vi "Write SV.vi"(8 "error in (no error)":errorcluster, 10 "Data":dbl[](array[numeric]), 11 "Write Refs by Type":T1) -> (0 "error out":errorcluster)   [LabVIEW 2016, in "Shared Variable Interface.lvlib"]
uses:
  Shared Variable Interface.lvlib
  DataTypes/DBL.lvlib
  DataTypes/Bool.lvlib
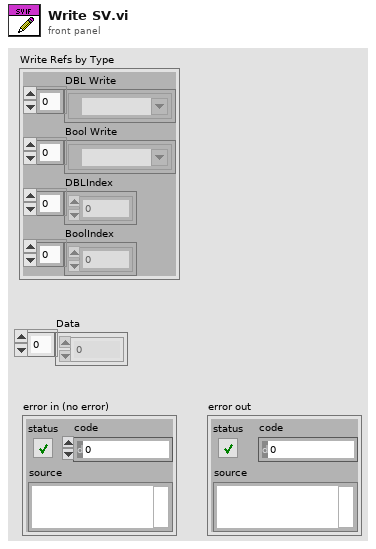
[diagram p1: front panel]
types:
  T1 = cluster{"DBL Write":refnum<k21>[], "Bool Write":refnum<k21>[], "DBLIndex":i32[], "BoolIndex":i32[]}
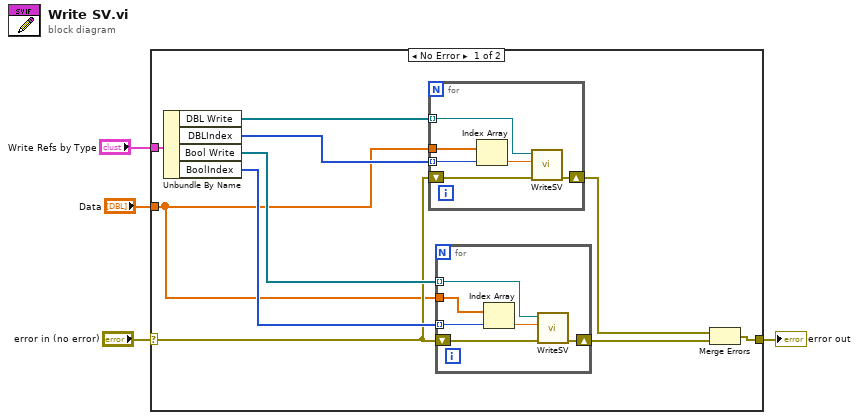
[diagram p0: block diagram]
diagram:
  n1 = case shown="No Error" "error in (no error)" {
    selector: "error in (no error)" -> [w7 w27]
    tunnel: [w14 w27] -> w4
    tunnel: "Data" -> [w6 _]
    tunnel: "Write Refs by Type" -> [w5 _]
    frame No Error {
      n2 = Unbundle By Name(w5) -> ("DBL Write"=w13:refnum<k21>[], "DBLIndex"=w12:i32[], "Bool Write"=w11:refnum<k21>[], "BoolIndex"=w10:i32[])
      n3 = for {
        tunnel: w13 -> [w21] mode=indexing
        tunnel: w12 -> [w26] mode=indexing
        shift-right: [w24] -> w8
        shift-left: w7 -> [w25]
        tunnel: w6 -> [w23]
        n4 = Index Array(array=w23, index=w26) -> (element=w22:dbl)
        n5 = call "WriteSV.vi"("error in (no error)"=w25, "DBL Data"=w22, "shared variable refnum in"=w21) -> ("error out"=w24:errorcluster)  [unwired: 8 in]
      }
      n6 = for {
        tunnel: w11 -> [w15] mode=indexing
        tunnel: w10 -> [w20] mode=indexing
        shift-right: [w17] -> w9
        shift-left: w7 -> [w18]
        tunnel: w6 -> [w19]
        n7 = Index Array(array=w19, index=w20) -> (element=w16:dbl)
        n8 = call "WriteSV.vi"("error in (no error)"=w18, "DBL Data"=w16, "shared variable refnum in"=w15) -> ("error out"=w17:errorcluster)  [unwired: 8 in]
      }
      n9 = Merge Errors(w8, w9) -> (w14:errorcluster)
    }
    frame Error {
    }
  }
  "error out" <- w4
